vi "Dequeue Message.vi"(8 "error in (no error)":errorcluster, 9 "timeout in ms (-1)":i32=-1, 11 "Process In":refnum<class "Process.lvclass">) -> (0 "error out":errorcluster, 1 "Message Data":variant, 2 "Message":string, 3 "Process Out":refnum<class "Process.lvclass">)   [LabVIEW 2020, in "Process.lvclass"]
doc: "This VI pulls messages off the Message Queue."
uses:
  Process.lvclass
  Process.lvclass/Process.ctl
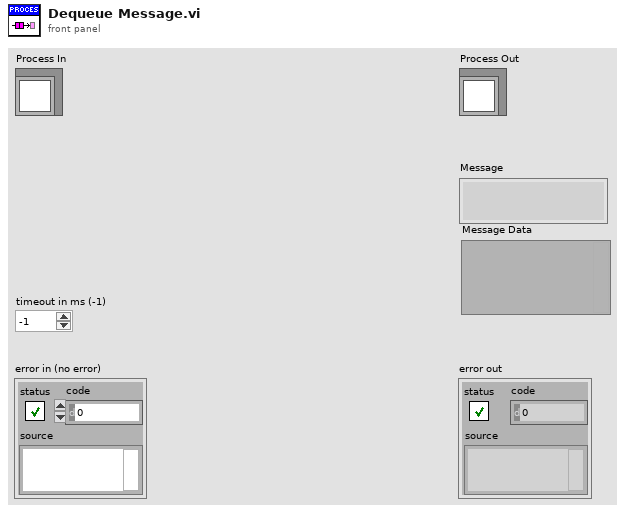
[diagram p1: front panel]
types:
  T1 = typedef "Process.lvclass/Message Cluster.ctl" = cluster{"Message":string, "Message Data":variant}
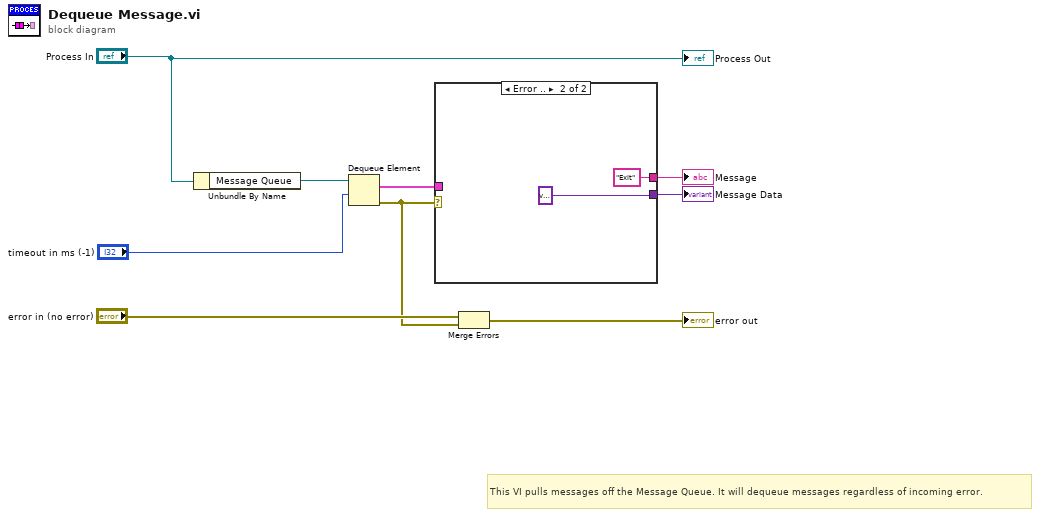
[diagram p0: block diagram]
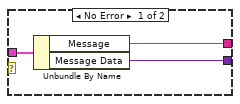
[diagram p2: hidden frame]
diagram:
  # "This VI pulls messages off the Message Queue. It will dequeue messages regardless of incoming error."
  n1 = Unbundle By Name("Process In") -> ("Message Queue"=w8:refnum<queue>)
  n2 = Dequeue Element(queue=w8, timeout in ms (-1)="timeout in ms (-1)") -> (element=w2:T1, error out=w1:errorcluster)  [unwired: 1 in, 2 out]
  n3 = case shown="Error .." w1 {
    tunnel: [w12 "Exit" ("Message")] -> w5
    tunnel: [w11 variant ("Message Data")] -> w4
    tunnel: w2 -> [w10 _]
    frame No Error {
      n4 = Unbundle By Name(w10) -> ("Message"=w12:string, "Message Data"=w11:variant)
    }
    frame Error {
    }
  }
  "Message" <- w5
  "Message Data" <- w4
  n5 = Merge Errors("error in (no error)", w1) -> (→"error out":errorcluster)
  "Process Out" <- "Process In"
